vi "Bounce(LC).vi"(0 "COMPORT":refnum<visa-resource-name>="COM4", 1 "i/q_file":string, 5 "Gui(path)":path=path "C:/RageATE-Tetra/Support/TetraLabGUI", 9 "Ft directory":path=path "C:/RageATE-Tetra/Support/FieldTestApp", 11 "error in (no error)":errorcluster, 12 "Controls":T1={"ReadADC"=TRUE, "StartTest"=TRUE, "ResetRFSM"=TRUE, "FtServer"=TRUE, "CalVCO(t)"=TRUE, "Ping(t)"=TRUE, "CmdWindowHide(T)"=FALSE, "OpenNewFt(T)"=TRUE, "UseCmdFile(T)"=FALSE}, 13 "Standalone vi(t)":bool, 14 "Write i/q data file":bool) -> (2 "PingOK?(t)":bool=TRUE, 3 "P/F Bounce":bool, 6 "Data_Out":string[][](array[string])=[["Index/Ant", "Tx_Ant", "Rx_Ant", "dBFS", "MHz", "P/F_Power", "P/F_Freq"], ["1", "1", "1", "-5.663", "-6.226", "PASS", "PASS"], ["2", "2", "1", "-7.008", "-6.226", "PASS", "PASS"], ["3", "1", "2", "-6.712", "-6.226", "PASS", "PASS"], ["4", "3", "1", "-7.302", "-6.226", "PASS", "PASS"], ["5", "2", "2", "-6.729", "-6.226", "PASS", "PASS"], ["6", "4", "1", "-7.411", "-6.226", "PASS", "PASS"], ["7", "3", "2", "-6.907", "-6.226", "PASS", "PASS"], ["8", "2", "3", "-5.919", "-6.152", "PASS", "PASS"], ["9", "4", "2", "-6.829", "-6.226", "PASS", "PASS"], ["10", "3", "3", "-5.795", "-6.226", "PASS", "PASS"], ["11", "5", "2", "-7.206", "-6.226", "PASS", "PASS"], ["12", "4", "3", "-6.209", "-6.226", "PASS", "PASS"], ["13", "3", "4", "-6.316", "-6.226", "PASS", "PASS"], ["14", "5", "3", "-5.848", "-6.226", "PASS", "PASS"], ["15", "4", "4", "-6.060", "-6.226", "PASS", "PASS"], ["16", "6", "3", "-6.797", "-6.226", "PASS", "PASS"], ["17", "5", "4", "-5.983", "-6.226", "PASS", "PASS"], ["18", "7", "3", "-5.772", "-6.152", "PASS", "PASS"], ["19", "6", "4", "-5.572", "-6.226", "PASS", "PASS"], ["20", "5", "5", "-6.223", "-6.226", "PASS", "PASS"], ["21", "7", "4", "-5.813", "-6.226", "PASS", "PASS"], ["22", "6", "5", "-6.423", "-6.226", "PASS", "PASS"], ["23", "8", "4", "-5.728", "-6.226", "PASS", "PASS"], ["24", "7", "5", "-5.739", "-6.226", "PASS", "PASS"], ["25", "6", "6", "-5.901", "-6.226", "PASS", "PASS"], ["26", "8", "5", "-5.879", "-6.226", "PASS", "PASS"], ["27", "7", "6", "-5.680", "-6.226", "PASS", "PASS"], ["28", "9", "5", "-6.898", "-6.226", "PASS", "PASS"], ["29", "8", "6", "-5.680", "-6.226", "PASS", "PASS"], ["30", "10", "5", "-6.902", "-6.226", "PASS", "PASS"], ["31", "9", "6", "-6.670", "-6.226", "PASS", "PASS"], ["32", "8", "7", "-5.577", "-6.226", "PASS", "PASS"], ["33", "10", "6", "-6.776", "-6.226", "PASS", "PASS"], ["34", "9", "7", "-6.721", "-6.226", "PASS", "PASS"], ["35", "11", "6", "-7.184", "-6.226", "PASS", "PASS"], ["36", "10", "7", "-7.166", "-6.226", "PASS", "PASS"], ["37", "9", "8", "-6.669", "-6.226", "PASS", "PASS"], ["38", "11", "7", "-6.752", "-6.226", "PASS", "PASS"], ["39", "10", "8", "-6.667", "-6.226", "PASS", "PASS"], ["40", "12", "7", "-6.185", "-6.226", "PASS", "PASS"], ["41", "11", "8", "-6.673", "-6.226", "PASS", "PASS"], ["42", "12", "8", "-7.339", "-6.226", "PASS", "PASS"]], 8 "Ampl_Graph":dbl[][](graph), 10 "Freq_Graph":dbl[](graph), 15 "error out":errorcluster)   [LabVIEW 2018]
uses:
  C:/RageATE-Tetra/Support/TetraLabGUI/FieldTestClient.dll
  Support/TetraLabGUI/FieldTestClient.dll
  Tetra WAM/Tetra_Globals.vi
panel:
  in  "Tab Control":enum32{"Gui", "Tabular", "Settings"}(tab)
  out "status":string
  out "RESULT:":string
  in  "START":bool
  in  "CONT(t)":bool
  out "Elapsed Time":string caption="Elapsed Time Text"
  in  "Rev-C(T)":bool
  out "#ofBounces":i32
  out "py_comport":string=" -COM4"
  in  "ampl_lsl":dbl=-12.5 format="%#_13g"
  in  "ampl_hsl":dbl=2.5 format="%#_13g"
  out "StartTest?(P/F)":bool
  out "VcoCalibration?(T)":bool
  out "Close":bool
  out "ReadADC":bool=TRUE
  out "StartTest":bool
  out "ResetRFSM":bool
  out "FtServer":bool
  out "CalVCO(t)":bool
  out "Ping(t)":bool=TRUE
  out "CmdWindowHide(T)":bool
  out "OpenNewFt(T)":bool
  out "UseCmdFile(T)":bool
  out "hostName":string="localhost"
  out "portNum":i32=50501
  out "standard output":string="b'OK\\n\\r'\r\nDMA Length: 43008\r\nTx_1 Rx_1: {'Frequency': 'Passed', 'Power': 'Passed'}\r\nMax Value: -5.663 dBFS at -6.226 MHz\r\nTx_2 Rx_1: {'Frequency': 'Passed', 'Power': 'Passed'}\r\nMax Value: -7.008 dBFS at -6.226 MHz\r\nTx_1 Rx_2: {'Frequency': 'Passed', 'Power': 'Passed'}\r\nMax Value: -6.712 dBFS at -6.226 MHz\r\nTx_3 Rx_1: {'Frequency': 'Passed', 'Power': 'Passed'}\r\nMax Value: -7.302 dBFS at -6.226 MHz\r\nTx_2 Rx_2: {'Frequency': 'Passed', 'Power': 'Passed'}\r\nMax Value: -6.729 dBFS at -6.226 MHz\r\nTx_4 Rx_1: {'Frequency': 'Passed', 'Power': 'Passed'}\r\nMax Value: -7.411 dBFS at -6.226 MHz\r\nTx_3 Rx_2: {'Frequency': 'Passed', 'Power': 'Passed'}\r\nMax Value: -6.907 dBFS at -6.226 MHz\r\nTx_2 Rx_3: {'Frequency': 'Passed', 'Power': 'Passed'}\r\nMax Value: -5.919 dBFS at -6.152 MHz\r\nTx_4 Rx_2: {'Frequency': 'Passed', 'Power': 'Passed'}\r\nMax Value: -6.829 dBFS at -6.226 MHz\r\nTx_3 Rx_3: {'Frequency': 'Passed', 'Power': 'Passed'}\r\nMax Value: -5.795 dBFS at -6.226 MHz\r\nTx_5 Rx_2: {'Frequency': 'Passed', 'Power': 'Passed'}\r\nMax Value: -7.206 dBFS at -6.226 MHz\r\nTx_4 Rx_3: {'Frequency': 'Passed', 'Power': 'Passed'}\r\nMax Value: -6.209 dBFS at -6.226 MHz\r\nTx_3 Rx_4: {'Frequency': 'Passed', 'Power': 'Passed'}\r\nMax Value: -6.316 dBFS at -6.226 MHz\r\nTx_5 Rx_3: {'Frequency': 'Passed', 'Power': 'Passed'}\r\nMax Value: -5.848 dBFS at -6.226 MHz\r\nTx_4 Rx_4: {'Frequency': 'Passed', 'Power': 'Passed'}\r\nMax Value: -6.060 dBFS at -6.226 MHz\r\nTx_6 Rx_3: {'Frequency': 'Passed', 'Power': 'Passed'}\r\nMax Value: -6.797 dBFS at -6.226 MHz\r\nTx_5 Rx_4: {'Frequency': 'Passed', 'Power': 'Passed'}\r\nMax Value: -5.983 dBFS at -6.226 MHz\r\nTx_7 Rx_3: {'Frequency': 'Passed', 'Power': 'Passed'}\r\nMax Value: -5.772 dBFS at -6.152 MHz\r\nTx_6 Rx_4: {'Frequency': 'Passed', 'Power': 'Passed'}\r\nMax Value: -5.572 dBFS at -6.226 MHz\r\nTx_5 Rx_5: {'Frequency': 'Passed', 'Power': 'Passed'}\r\nMax Value: -6.223 dBFS at -6.226 MHz\r\nTx_7 Rx_4: {'Frequency': 'Passed', 'Power': 'Passed'}\r\nMax Value: -5.813 dBFS at -6.226 MHz\r\nTx_6 Rx_5: {'Frequency': 'Passed', 'Power': 'Passed'}\r\nMax Value: -6.423 dBFS at -6.226 MHz\r\nTx_8 Rx_4: {'Frequency': 'Passed', 'Power': 'Passed'}\r\nMax Value: -5.728 dBFS at -6.226 MHz\r\nTx_7 Rx_5: {'Frequency': 'Passed', 'Power': 'Passed'}\r\nMax Value: -5.739 dBFS at -6.226 MHz\r\nTx_6 Rx_6: {'Frequency': 'Passed', 'Power': 'Passed'}\r\nMax Value: -5.901 dBFS at -6.226 MHz\r\nTx_8 Rx_5: {'Frequency': 'Passed', 'Power': 'Passed'}\r\nMax Value: -5.879 dBFS at -6.226 MHz\r\nTx_7 Rx_6: {'Frequency': 'Passed', 'Power': 'Passed'}\r\nMax Value: -5.680 dBFS at -6.226 MHz\r\nTx_9 Rx_5: {'Frequency': 'Passed', 'Power': 'Passed'}\r\nMax Value: -6.898 dBFS at -6.226 MHz\r\nTx_8 Rx_6: {'Frequency': 'Passed', 'Power': 'Passed'}\r\nMax Value: -5.680 dBFS at -6.226 MHz\r\nTx_10 Rx_5: {'Frequency': 'Passed', 'Power': 'Passed'}\r\nMax Value: -6.902 dBFS at -6.226 MHz\r\nTx_9 Rx_6: {'Frequency': 'Passed', 'Power': 'Passed'}\r\nMax Value: -6.670 dBFS at -6.226 MHz\r\nTx_8 Rx_7: {'Frequency': 'Passed', 'Power': 'Passed'}\r\nMax Value: -5.577 dBFS at -6.226 MHz\r\nTx_10 Rx_6: {'Frequency': 'Passed', 'Power': 'Passed'}\r\nMax Value: -6.776 dBFS at -6.226 MHz\r\nTx_9 Rx_7: {'Frequency': 'Passed', 'Power': 'Passed'}\r\nMax Value: -6.721 dBFS at -6.226 MHz\r\nTx_11 Rx_6: {'Frequency': 'Passed', 'Power': 'Passed'}\r\nMax Value: -7.184 dBFS at -6.226 MHz\r\nTx_10 Rx_7: {'Frequency': 'Passed', 'Power': 'Passed'}\r\nMax Value: -7.166 dBFS at -6.226 MHz\r\nTx_9 Rx_8: {'Frequency': 'Passed', 'Power': 'Passed'}\r\nMax Value: -6.669 dBFS at -6.226 MHz\r\nTx_11 Rx_7: {'Frequency': 'Passed', 'Power': 'Passed'}\r\nMax Value: -6.752 dBFS at -6.226 MHz\r\nTx_10 Rx_8: {'Frequency': 'Passed', 'Power': 'Passed'}\r\nMax Value: -6.667 dBFS at -6.226 MHz\r\nTx_12 Rx_7: {'Frequency': 'Passed', 'Power': 'Passed'}\r\nMax Value: -6.185 dBFS at -6.226 MHz\r\nTx_11 Rx_8: {'Frequency': 'Passed', 'Power': 'Passed'}\r\nMax Value: -6.673 dBFS at -6.226 MHz\r\nTx_12 Rx_8: {'Frequency': 'Passed', 'Power': 'Passed'}\r\nMax Value: -7.339 dBFS at -6.226 MHz\r\n"
  out "standard error":string
  out "ReadADC_Command":string
  out "ref_time":dbl caption="Get Start Time (s)"
  out "AMPL(P/F)":bool
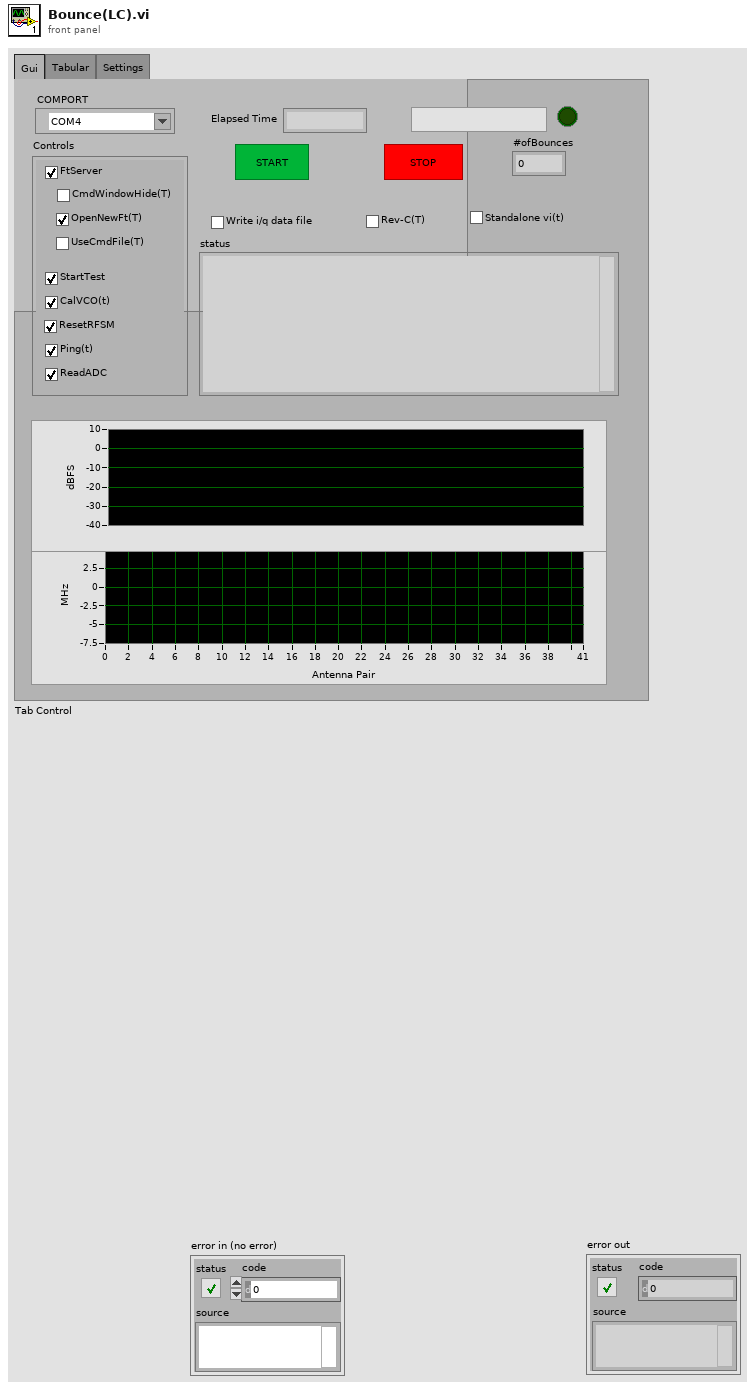
[diagram p1: front panel]
types:
  T1 = cluster{"ReadADC":bool, "StartTest":bool, "ResetRFSM":bool, "FtServer":bool, "CalVCO(t)":bool, "Ping(t)":bool, "CmdWindowHide(T)":bool, "OpenNewFt(T)":bool, "UseCmdFile(T)":bool}
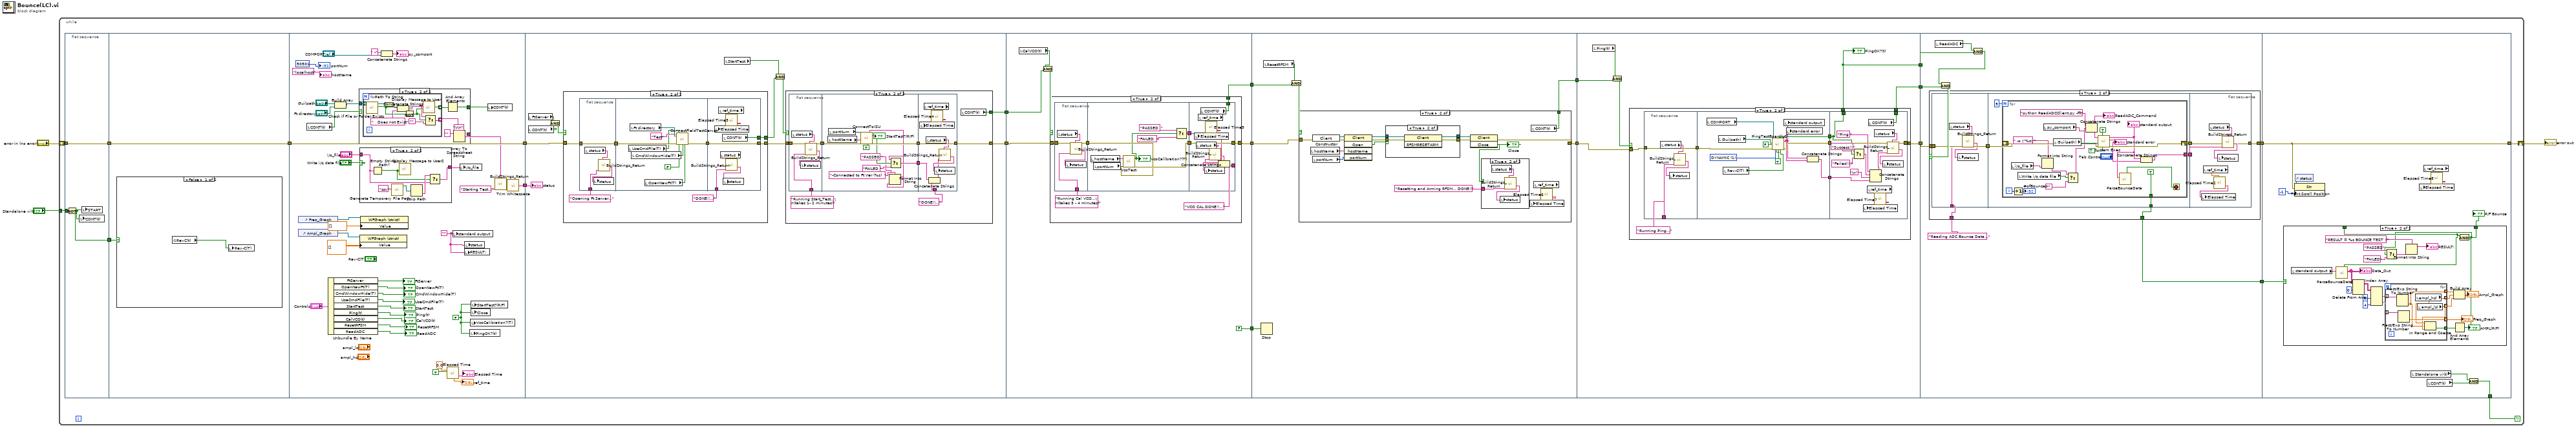
[diagram p0: block diagram]
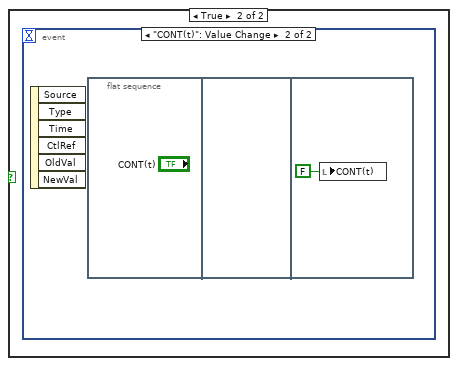
[diagram p2: hidden frame]
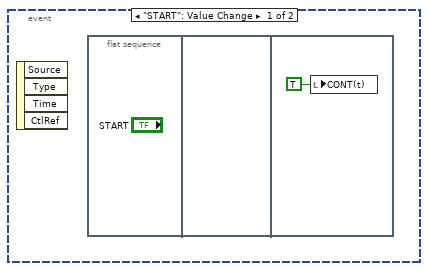
[diagram p3: hidden frame]
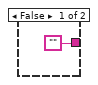
[diagram p4: hidden frame]
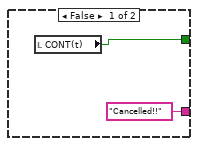
[diagram p5: hidden frame]
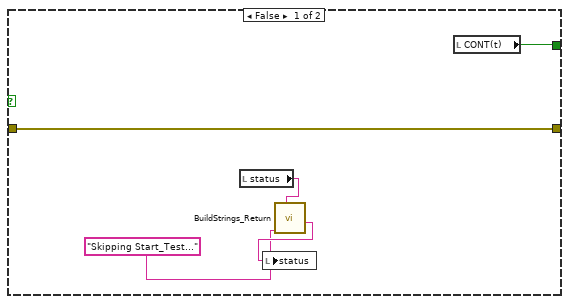
[diagram p6: hidden frame]
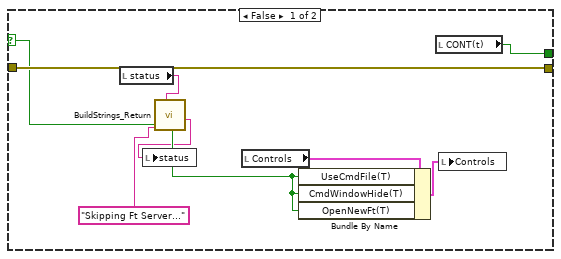
[diagram p7: hidden frame]
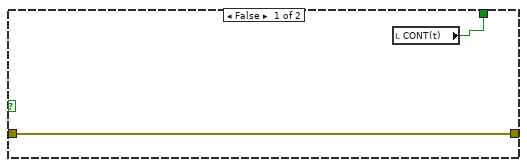
[diagram p8: hidden frame]
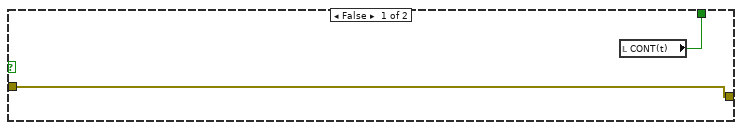
[diagram p9: hidden frame]
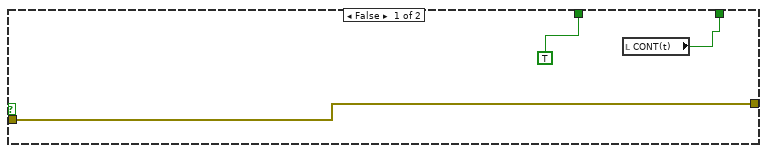
[diagram p12: hidden frame]
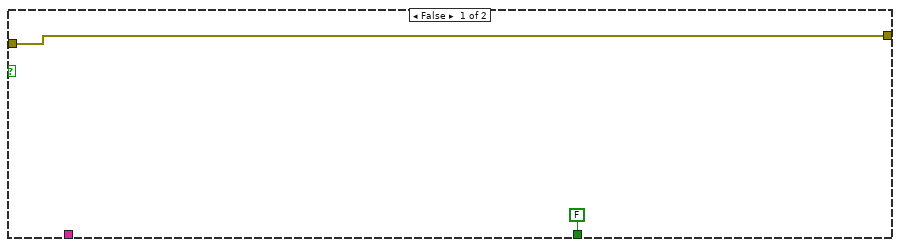
[diagram p13: hidden frame]
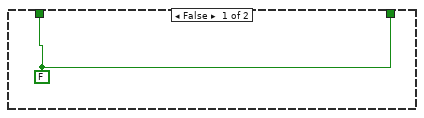
[diagram p14: hidden frame]
diagram:
  n1 = while {
    shift-right: [w14] -> w2
    shift-left: "error in (no error)" -> [w15]
    tunnel: "Standalone vi(t)" -> [w5]
    stop <- w11 continue-if-true
    n2 = flat-sequence {
      tunnel: w15 -> [w27]
      tunnel: [w27] -> w12
      tunnel: w5 -> [w25]
      tunnel: [w25] -> w4
      tunnel: [w29] -> w13
      tunnel: w12 -> [w29]
      tunnel: w4 -> [w28]
      tunnel: [w70] -> w24
      tunnel: [w61] -> w23
      tunnel: w13 -> [w70]
      tunnel: [w103] -> w22
      tunnel: w24 -> [w105]
      tunnel: w23 -> [w104]
      tunnel: [w95] -> w9
      tunnel: w22 -> [w183]
      tunnel: [w182] -> w21
      tunnel: [FALSE ("stop? (T)")] -> w10
      tunnel: w9 -> [w178]
      tunnel: [w177] -> w8
      tunnel: w21 -> [w221]
      tunnel: [w220] -> w20
      tunnel: w10 -> [w218]
      tunnel: w8 -> [w216]
      tunnel: [w215] -> w7
      tunnel: [w255] -> w18
      tunnel: w20 -> [w254]
      tunnel: [w253] -> w19
      tunnel: w7 -> [w250]
      tunnel: [w249] -> w6
      tunnel: w19 -> [w304]
      tunnel: w18 -> [w305]
      tunnel: [w306] -> w17
      tunnel: [w301] -> w16
      tunnel: w6 -> [w298]
      tunnel: [w359] -> w14
      tunnel: w17 -> [w359]
      tunnel: w16 -> [w358]
      tunnel: [w354] -> w11
      frame #0 {
        n3 = Not(x=w25) -> (.not. x?=w26:bool)
        n4 = local write "CONT(t)"(w26) -> ()
        n5 = local write "START"(w26) -> ()
      }
      frame #1 {
        n6 = case shown="False" w28 {
          frame False {
            n7 = global read "Tetra_Globals.vi" "RevC(t)"() -> (w30:bool)
            n8 = local write "Rev-C(T)"(w30) -> ()
          }
          frame True {
            n9 = event shown="[1] \"CONT(t)\": Value Change" {
              selector: _ -> [_ _]
              dyn-events: _ -> [_ _]
              timeout: _ -> [_ _]
              event "START": Value Change {
                n10 = event-data() -> ()  [unwired: 1 in, 4 out]
                n11 = flat-sequence {
                  frame #0 {
                  }
                  frame #1 {
                  }
                  frame #2 {
                    n12 = local write "CONT(t)"(TRUE ("CONT(t)")) -> ()
                  }
                }
              }
              event "CONT(t)": Value Change {
                n13 = event-data() -> ()  [unwired: 1 in, 6 out]
                n14 = flat-sequence {
                  frame #0 {
                  }
                  frame #1 {
                  }
                  frame #2 {
                    n15 = local write "CONT(t)"(FALSE ("CONT(t)")) -> ()
                  }
                }
              }
            }
          }
        }
      }
      frame #2 {
        w67 = FALSE ("StartTest?(P/F)")
        w49 = ""
        n16 = control-ref of="Ampl_Graph"() -> (w60:refnum<vi>)
        n17 = control-ref of="Freq_Graph"() -> (w59:refnum<vi>)
        n18 = local read "CONT(t)"() -> (w38:bool)
        n19 = Unbundle By Name("Controls") -> ("FtServer"=→"FtServer":bool, "OpenNewFt(T)"=→"OpenNewFt(T)":bool, "CmdWindowHide(T)"=→"CmdWindowHide(T)":bool, "UseCmdFile(T)"=→"UseCmdFile(T)":bool, "StartTest"=→"StartTest":bool, "Ping(t)"=→"Ping(t)":bool, "CalVCO(t)"=→"CalVCO(t)":bool, "ResetRFSM"=→"ResetRFSM":bool, "ReadADC"=→"ReadADC":bool)
        n20 = Build Array("Gui(path)", "Ft directory") -> (w42:path[])
        n21 = case shown="True" w38 {
          tunnel: w42 -> [_ w86]
          tunnel: [w79 w84] -> w40
          tunnel: ["Cancelled!!" ("spreadsheet string") w83] -> w39
          frame False {
            n22 = local read "CONT(t)"() -> (w79:bool)
          }
          frame True {
            n23 = for {
              tunnel: w86 -> [w94] mode=indexing
              tunnel: [w87] -> w85 mode=indexing
              tunnel: [w88] -> w82 mode=indexing
              n24 = call <vilib>:"Check if File or Folder Exists.vi"("path"=w94) -> ("file or folder exists?"=w87:bool)  [unwired: 8 in, 2 out]
              n25 = Path To String(path=w94) -> (string=w93:string)
              n26 = Concatenate Strings(w93, "   Does not Exist" ("string")) -> (w90:string)
              n27 = Not(x=w87) -> (.not. x?=w91:bool)
              n28 = call "Display Message to User"("Enable"=w91, "Message"=w90) -> ()  [unwired: 8 in, 2 out]
              n29 = Select(t=w90, s=w91, f="") -> (s? t:f=w88:string)
            }
            n30 = And Array Elements(Boolean array=w85) -> (logical AND=w84:bool)
            n31 = Array To Spreadsheet String(delimiter (Tab)="\r\n", array=w82, 3:"" ("format string")) -> (spreadsheet string=w83:string)
          }
        }
        n32 = case shown="True" "Write i/q data file" {
          tunnel: ["" w75] -> w34
          tunnel: "i/q_file" -> [_ w73]
          frame False {
          }
          frame True {
            n33 = Empty String/Path?(string/path=w73) -> (empty?=w72:bool)
            n34 = call <vilib>:"Generate Temporary File Path.vi"("Temporary File Extension (tmp)"="csv") -> ("Unique Temporary File Path"=w76:path)  [unwired: 9 in, 1 out]
            n35 = call "Display Message to User2"("Enable"=w72) -> ()  [unwired: 9 in, 2 out]
            n36 = Strip Path(path=w76) -> (name=w74:string)  [unwired: 1 out]
            n37 = Select(t=w74, s=w72, f=w73) -> (s? t:f=w75:string)
          }
        }
        n38 = property class="WFGraph (strict)"(reference=w60, "Value"=dbl[][] []) -> ()  [unwired: 1 in, 2 out]
        n39 = property class="WFGraph (strict)"(reference=w59, "Value"=dbl[] []) -> ()  [unwired: 1 in, 2 out]
        n40 = Concatenate Strings(" -" ("string"), "COMPORT") -> (→"py_comport":string)
        n41 = call "Elapsed Time"("Reset"=TRUE, "Set Start Time (s)"=0.0) -> ("Get Start Time (s)"=→"ref_time":dbl, "Elapsed Time Text"=→"Elapsed Time":string)  [unwired: 10 in, 6 out]
        n42 = local write "standard output"(w49) -> ()
        n43 = local write "i/q_file"(w34) -> ()
        n44 = local write "RESULT:"(w49) -> ()
        n45 = local write "status"(w49) -> ()
        n46 = local write "PingOK?(t)"(w67) -> ()
        n47 = local write "VcoCalibration?(T)"(w67) -> ()
        n48 = local write "StartTest?(P/F)"(w67) -> ()
        n49 = local write "Close"(w67) -> ()
        n50 = local write "CONT(t)"(w40) -> ()
        n51 = call "BuildStrings_Return.vi"("Input String"=w39, "New String"="Starting Test...") -> ("concatenated string"=w62:string)  [unwired: 7 in, 2 out]
        n52 = call <vilib>:"Trim Whitespace.vi"("string"=w62) -> ("trimmed string"=w61:string)  [unwired: 1 in]
        "hostName" <- "localhost" ("hostName")
        "portNum" <- 50501 ("portNum")
      }
      frame #3 {
        n53 = local read "FtServer"() -> (w101:bool)
        n54 = local read "CONT(t)"() -> (w99:bool)
        n55 = And(x=w101, y=w99) -> (x .and. y?=w100:bool)
        n56 = case shown="True" w100 {
          selector: w100 -> [w147 _]
          tunnel: w105 -> [w150 w157]
          tunnel: [w150 w156] -> w102
          tunnel: [w143 w151] -> w96
          frame False {
            n57 = local read "status"() -> (w146:string)
            n58 = call "BuildStrings_Return.vi"("Input String"=w146, "New String"="Skipping Ft Server...") -> ("concatenated string"=w145:string)  [unwired: 7 in, 2 out]
            n59 = local write "status"(w145) -> ()
            n60 = local read "Controls"() -> (w149:T1)
            n61 = Bundle By Name(cluster=w149, "UseCmdFile(T)"=w147, "CmdWindowHide(T)"=w147, "OpenNewFt(T)"=w147) -> (w148:T1)
            n62 = local read "CONT(t)"() -> (w143:bool)
            n63 = local write "Controls"(w148) -> ()
          }
          frame True {
            n64 = flat-sequence {
              tunnel: w157 -> [w161]
              tunnel: [w161] -> w154
              tunnel: "Opening Ft Server..." -> [w159]
              tunnel: [w168] -> w155
              tunnel: w154 -> [w169]
              tunnel: [w176] -> w156
              tunnel: w155 -> [w176]
              tunnel: "DONE!!..." -> [w174]
              tunnel: [w170] -> w151
              frame #0 {
                n65 = local read "status"() -> (w160:string)
                n66 = call "BuildStrings_Return.vi"("Input String"=w160, "New String"=w159) -> ("concatenated string"=w158:string)  [unwired: 7 in, 2 out]
                n67 = local write "status"(w158) -> ()
              }
              frame #1 {
                n68 = local read "UseCmdFile(T)"() -> (w162:bool)
                n69 = local read "Ft directory"() -> (w167:path)
                n70 = local read "CmdWindowHide(T)"() -> (w163:bool)
                n71 = local read "OpenNewFt(T)"() -> (w164:bool)
                n72 = call "ConnectFieldTestServer.vi"("FileName(.txt)"="Test", "working directory"=w167, "error in (no error)"=w169, "UseCmdFile(T)"=w162, "Skip(T)"=FALSE, "CmdWindowHide(T)"=w163, "OpenNewFt(T)"=w164) -> ("error out"=w168:errorcluster)  [unwired: 6 in, 6 out]
              }
              frame #2 {
                n73 = local read "ref_time"() -> (w171:dbl)
                n74 = local read "status"() -> (w175:string)
                n75 = local read "CONT(t)"() -> (w170:bool)
                n76 = call "Elapsed Time3"("Set Start Time (s)"=w171) -> ("Elapsed Time Text"=w172:string)  [unwired: 11 in, 7 out]
                n77 = local write "Elapsed Time"(w172) -> ()
                n78 = call "BuildStrings_Return.vi"("Input String"=w175, "New String"=w174) -> ("concatenated string"=w173:string)  [unwired: 7 in, 2 out]
                n79 = local write "status"(w173) -> ()
              }
            }
          }
        }
        n80 = local read "StartTest"() -> (w98:bool)
        n81 = And(x=w98, y=w96) -> (x .and. y?=w97:bool)
        n82 = case shown="True" w97 {
          tunnel: w102 -> [w110 w118]
          tunnel: [w110 w117] -> w103
          tunnel: [w106 w111] -> w95
          frame False {
            n83 = local read "status"() -> (w108:string)
            n84 = call "BuildStrings_Return.vi"("Input String"=w108, "New String"="Skipping Start_Test...") -> ("concatenated string"=w109:string)  [unwired: 7 in, 2 out]
            n85 = local write "status"(w109) -> ()
            n86 = local read "CONT(t)"() -> (w106:bool)
          }
          frame True {
            n87 = flat-sequence {
              tunnel: w118 -> [w122]
              tunnel: [w122] -> w116
              tunnel: "Running Start_Test...\n(takes 1- 2 minutes)" -> [w119]
              tunnel: w116 -> [w134]
              tunnel: [w133] -> w115
              tunnel: [w127] -> w112
              tunnel: [w142] -> w117
              tunnel: w115 -> [w142]
              tunnel: "DONE!!..." -> [w139]
              tunnel: w112 -> [w137]
              frame #0 {
                n88 = local read "status"() -> (w121:string)
                n89 = call "BuildStrings_Return.vi"("Input String"=w121, "New String"=w119) -> ("concatenated string"=w120:string)  [unwired: 7 in, 2 out]
                n90 = local write "status"(w120) -> ()
              }
              frame #1 {
                n91 = local read "hostName"() -> (w131:string)
                n92 = local read "portNum"() -> (w132:i32)
                n93 = call "ConnectToISU.vi"("error in (no error)"=w134, "hostName"=w131, "portNum"=w132, "RunStartTest(T)"=TRUE) -> ("StartTest?(P/F)"=w128:bool, "GetVersion"=w124:string, "error out"=w133:errorcluster)  [unwired: 11 in, 2 out]
                "StartTest?(P/F)" <- w128
                n94 = Format Into String(format string="-Connected to Ft Ver (%s)  ", initial string="PASSED ", w124) -> (resulting string=w123:string)  [unwired: 1 in, 1 out]
                n95 = Select(t=w123, s=w128, f="FAILED ") -> (s? t:f=w127:string)
              }
              frame #2 {
                n96 = local read "ref_time"() -> (w135:dbl)
                n97 = local read "status"() -> (w140:string)
                n98 = Concatenate Strings(w137, w139) -> (w138:string)
                n99 = call "Elapsed Time4"("Set Start Time (s)"=w135) -> ("Elapsed Time Text"=w136:string)  [unwired: 11 in, 7 out]
                n100 = local write "Elapsed Time"(w136) -> ()
                n101 = call "BuildStrings_Return.vi"("Input String"=w140, "New String"=w138) -> ("concatenated string"=w141:string)  [unwired: 7 in, 2 out]
                n102 = local write "status"(w141) -> ()
              }
            }
            n103 = local read "CONT(t)"() -> (w111:bool)
          }
        }
        "status" <- w104
      }
      frame #4 {
        n104 = local read "CalVCO(t)"() -> (w181:bool)
        n105 = And(x=w181, y=w178) -> (x .and. y?=w179:bool)
        n106 = case shown="True" w179 {
          tunnel: w183 -> [w185 w193]
          tunnel: [w185 w192] -> w182
          tunnel: [w184 w186] -> w177
          frame False {
            n107 = local read "CONT(t)"() -> (w184:bool)
          }
          frame True {
            n108 = flat-sequence {
              tunnel: w193 -> [w197]
              tunnel: [w197] -> w191
              tunnel: "Running Cal VCO...\n(takes 3 - 4 minutes)" -> [w194]
              tunnel: w191 -> [w202]
              tunnel: [w203] -> w190
              tunnel: [w198] -> w187
              tunnel: [w214] -> w192
              tunnel: w190 -> [w214]
              tunnel: "VCO CAL DONE!!..." -> [w211]
              tunnel: w187 -> [w209]
              tunnel: [w206] -> w186
              frame #0 {
                n109 = local read "status"() -> (w196:string)
                n110 = call "BuildStrings_Return.vi"("Input String"=w196, "New String"=w194) -> ("concatenated string"=w195:string)  [unwired: 7 in, 2 out]
                n111 = local write "status"(w195) -> ()
              }
              frame #1 {
                n112 = local read "hostName"() -> (w205:string)
                n113 = local read "portNum"() -> (w204:i32)
                n114 = call "VcoTest.vi"("error in (no error)"=w202, "hostName"=w205, "portNum"=w204) -> ("VcoCalibration?(T)"=w199:bool, "error out"=w203:errorcluster)  [unwired: 13 in, 2 out]
                "VcoCalibration?(T)" <- w199
                n115 = Select(t="PASSED  ", s=w199, f="FAILED  ") -> (s? t:f=w198:string)
              }
              frame #2 {
                n116 = local read "status"() -> (w212:string)
                n117 = local read "ref_time"() -> (w207:dbl)
                n118 = local read "CONT(t)"() -> (w206:bool)
                n119 = call "Elapsed Time5"("Set Start Time (s)"=w207) -> ("Elapsed Time Text"=w208:string)  [unwired: 11 in, 7 out]
                n120 = local write "Elapsed Time"(w208) -> ()
                n121 = Concatenate Strings(w209, w211) -> (w210:string)
                n122 = call "BuildStrings_Return.vi"("Input String"=w212, "New String"=w210) -> ("concatenated string"=w213:string)  [unwired: 7 in, 2 out]
                n123 = local write "status"(w213) -> ()
              }
            }
          }
        }
      }
      frame #5 {
        n124 = Stop(stop? (T)=w218) -> ()
        n125 = local read "ResetRFSM"() -> (w219:bool)
        n126 = And(x=w219, y=w216) -> (x .and. y?=w217:bool)
        n127 = case shown="True" w217 {
          tunnel: w221 -> [w223 w239]
          tunnel: [w223 w227] -> w220
          tunnel: [w222 w224] -> w215
          frame False {
            n128 = local read "CONT(t)"() -> (w222:bool)
          }
          frame True {
            n129 = local read "hostName"() -> (w237:string)
            n130 = constructor class="Client"(error in=w239) -> (reference out=w238:refnum<k24>, error out=w234:errorcluster)  [unwired: 2 in, 1 out]
            n131 = local read "portNum"() -> (w236:i32)
            n132 = invoke class="Client" method="Open"(reference=w238, error in=w234, "hostName"=w237, "portNum"=w236) -> (reference out=w235:refnum<k24>, error out=w233:errorcluster, "Open"=w232:bool)  [unwired: 1 in, 2 out]
            n133 = case shown="True" w232 {
              tunnel: [w244 w248] -> w230
              tunnel: w235 -> [w243 w246]
              tunnel: w233 -> [w244 w245]
              tunnel: [w243 w247] -> w231
              frame False {
              }
              frame True {
                n134 = invoke class="Client" method="RFSMRESETARM"(reference=w246, error in=w245) -> (reference out=w247:refnum<k24>, error out=w248:errorcluster)  [unwired: 1 in, 1 out]
              }
            }
            n135 = invoke class="Client" method="Close"(reference=w231, error in=w230) -> (error out=w227:errorcluster, "Close"=w228:bool)  [unwired: 1 in, 1 out]
            "Close" <- w228
            n136 = case shown="True" w228 {
              tunnel: "Resetting and Arming RFSM... DONE!!" -> [_ w240]
              frame False {
              }
              frame True {
                n137 = local read "status"() -> (w242:string)
                n138 = call "BuildStrings_Return.vi"("Input String"=w242, "New String"=w240) -> ("concatenated string"=w241:string)  [unwired: 7 in, 2 out]
                n139 = local write "status"(w241) -> ()
              }
            }
            n140 = local read "CONT(t)"() -> (w224:bool)
            n141 = local read "ref_time"() -> (w226:dbl)
            n142 = call "Elapsed Time6"("Set Start Time (s)"=w226) -> ("Elapsed Time Text"=w225:string)  [unwired: 11 in, 7 out]
            n143 = local write "Elapsed Time"(w225) -> ()
          }
        }
      }
      frame #6 {
        n144 = local read "Ping(t)"() -> (w252:bool)
        n145 = And(x=w252, y=w250) -> (x .and. y?=w251:bool)
        n146 = case shown="True" w251 {
          tunnel: [w258 w260] -> w255
          tunnel: w254 -> [w258 w267]
          tunnel: [TRUE ("OK?(t)") w262] -> w253
          tunnel: [w256 w259] -> w249
          frame False {
            n147 = local read "CONT(t)"() -> (w256:bool)
          }
          frame True {
            n148 = flat-sequence {
              tunnel: w267 -> [w271]
              tunnel: [w271] -> w265
              tunnel: "Running Ping..." -> [w268]
              tunnel: [w283] -> w266
              tunnel: w265 -> [w282]
              tunnel: [w277] -> w263
              tunnel: [w274] -> w261
              tunnel: [w297] -> w260
              tunnel: w266 -> [w297]
              tunnel: w263 -> [w294]
              tunnel: [w294] -> w262
              tunnel: w261 -> [w289]
              tunnel: [w284] -> w259
              frame #0 {
                n149 = local read "status"() -> (w269:string)
                n150 = call "BuildStrings_Return.vi"("Input String"=w269, "New String"=w268) -> ("concatenated string"=w270:string)  [unwired: 7 in, 2 out]
                n151 = local write "status"(w270) -> ()
              }
              frame #1 {
                w280 = TRUE ("ExeCommands(T)")
                w281 = 1 items=["CW", "DYNAMIC"] ("Mode Select")
                n152 = local read "COMPORT"() -> (w278:refnum<visa-resource-name>)
                n153 = local read "Gui(path)"() -> (w279:path)
                n154 = local read "Rev-C(T)"() -> (w272:bool)
                n155 = call "PingTestBoard(LC).vi"("COMPORT"=w278, "GuiDir"=w279, "GlobPaths(t)"=FALSE, "error in (no error)"=w282, "Mode Select"=w281, "Close Serial(T)"=w280, "ExeCommands(T)"=w280, "RevC(t)"=w272) -> ("standard error"=w275:string, "standard output"=w276:string, "OK?(t)"=w277:bool, "error out"=w283:errorcluster)  [unwired: 5 in, 3 out]
                n156 = local write "standard output"(w276) -> ()
                n157 = local write "standard error"(w275) -> ()
                n158 = Concatenate Strings(w276, w275) -> (w274:string)
              }
              frame #2 {
                n159 = Select(t="Success!! ", s=w294, f="Failed!! ") -> (s? t:f=w292:string)
                n160 = local read "ref_time"() -> (w285:dbl)
                n161 = local read "CONT(t)"() -> (w284:bool)
                n162 = Concatenate Strings("Ping ", w292, "\n", w289) -> (w287:string)
                n163 = local read "status"() -> (w296:string)
                n164 = call "Elapsed Time7"("Set Start Time (s)"=w285) -> ("Elapsed Time Text"=w286:string)  [unwired: 11 in, 7 out]
                n165 = local write "Elapsed Time"(w286) -> ()
                n166 = call "BuildStrings_Return.vi"("Input String"=w296, "New String"=w287) -> ("concatenated string"=w295:string)  [unwired: 7 in, 2 out]
                n167 = local write "status"(w295) -> ()
              }
            }
          }
        }
        "PingOK?(t)" <- w253
      }
      frame #7 {
        n168 = local read "ReadADC"() -> (w302:bool)
        n169 = And(x=w302, y=w304) -> (x .and. y?=w300:bool)
        n170 = And(x=w300, y=w298) -> (x .and. y?=w299:bool)
        n171 = case shown="True" w299 {
          tunnel: [w307 w312] -> w306
          tunnel: w305 -> [w307 w311]
          tunnel: "Reading ADC Bounce Data..." -> [_ w310]
          tunnel: [FALSE w309] -> w301
          frame False {
          }
          frame True {
            n172 = flat-sequence {
              tunnel: w311 -> [w319]
              tunnel: [w319] -> w315
              tunnel: w310 -> [w316]
              tunnel: w315 -> [w323]
              tunnel: [w324] -> w314
              tunnel: [w322] -> w313
              tunnel: [w321] -> w309
              tunnel: [w348] -> w312
              tunnel: w314 -> [w348]
              tunnel: w313 -> [w349]
              frame #0 {
                n173 = local read "status"() -> (w318:string)
                n174 = call "BuildStrings_Return.vi"("Input String"=w318, "New String"=w316) -> ("concatenated string"=w317:string)  [unwired: 7 in, 2 out]
                n175 = local write "status"(w317) -> ()
              }
              frame #1 {
                n176 = for {
                  N: 5 -> [_]
                  tunnel: [w343] -> w322
                  tunnel: [TRUE] -> w321
                  shift-right: [w345] -> w324
                  shift-left: w323 -> [w344]
                  i -> [w326]
                  stop <- w328 stop-if-true
                  n177 = local read "i/q_file"() -> (w331:string)
                  n178 = Increment(x=w326) -> (x+1=→"#ofBounces":i32)
                  n179 = local read "Write i/q data file"() -> (w335:bool)
                  n180 = Format Into String(format string=" -o \"%s\"", w331) -> (resulting string=w332:string)  [unwired: 2 in, 1 out]
                  n181 = local read "py_comport"() -> (w329:string)
                  n182 = local read "Gui(path)"() -> (w338:path)
                  n183 = Select(t=w332, s=w335, f="") -> (s? t:f=w330:string)
                  n184 = Concatenate Strings("python ReadADCClient.py -fft" ("command line 3"), w330, w329) -> (w337:string)
                  "ReadADC_Command" <- w337
                  n185 = call <vilib>:"System Exec.vi"("run minimized? (F)"=TRUE, "wait until completion? (T)"=TRUE, "error in (no error)"=w344, "working directory"=w338, "command line"=w337) -> ("error out"=w345:errorcluster, "standard error"=w336:string, "standard output"=w327:string)  [unwired: 3 in, 1 out]
                  "standard error" <- w336
                  "standard output" <- w327
                  n186 = call "ParseBounceData.vi"("Data_In"=w327) -> ("Passed?(T)"=w328:bool)  [unwired: 12 in, 2 out]
                  n187 = Concatenate Strings(w327, w336) -> (w343:string)
                }
              }
              frame #2 {
                n188 = local read "ref_time"() -> (w346:dbl)
                n189 = local read "status"() -> (w350:string)
                n190 = call "Elapsed Time2"("Set Start Time (s)"=w346) -> ("Elapsed Time Text"=w347:string)  [unwired: 11 in, 7 out]
                n191 = local write "Elapsed Time"(w347) -> ()
                n192 = call "BuildStrings_Return.vi"("Input String"=w350, "New String"=w349) -> ("concatenated string"=w351:string)  [unwired: 7 in, 2 out]
                n193 = local write "status"(w351) -> ()
              }
            }
          }
        }
      }
      frame #8 {
        n194 = case shown="True" w358 {
          tunnel: [w362 w364] -> _
          tunnel: [w362 w363] -> w352
          frame False {
            w362 = FALSE ("Passed?(T)")
          }
          frame True {
            n195 = local read "standard output"() -> (w384:string)
            n196 = call "ParseBounceData.vi"("Data_In"=w384) -> ("Passed?(T)"=w364:bool, "Data_Out"=w382:string[][])  [unwired: 12 in, 1 out]
            "Data_Out" <- w382
            n197 = Delete From Array(array=w382, index (row)=0) -> (array with subset deleted=w380:string[][])  [unwired: 2 in, 1 out]
            n198 = Index Array(array=w380, index (col) #1=3 ("index (col)"), index (col) #2=4 ("index (col)")) -> (element #1=w379:string[], element #2=w376:string[])  [unwired: 2 in]
            n199 = for {
              tunnel: w379 -> [w391] mode=indexing
              tunnel: [w386] -> w378 mode=indexing
              tunnel: w376 -> [w390] mode=indexing
              tunnel: [w389] -> w375 mode=indexing
              tunnel: [w388] -> w368 mode=indexing
              tunnel: [w387] -> w367 mode=indexing
              tunnel: [w385] -> w366 mode=indexing
              n200 = Fract/Exp String To Number(string=w391) -> (number=w386:dbl)  [unwired: 3 in, 1 out]
              n201 = Fract/Exp String To Number(string=w390) -> (number=w389:dbl)  [unwired: 3 in, 1 out]
              n202 = local read "ampl_hsl"() -> (w388:dbl)
              n203 = local read "ampl_lsl"() -> (w387:dbl)
              n204 = In Range and Coerce(upper limit=w388, x=w386, lower limit=w387) -> (In Range?=w385:bool)  [unwired: 1 out]
            }
            "Freq_Graph" <- w375
            n205 = Build Array(w378, w368, w367) -> (→"Ampl_Graph":dbl[][])
            n206 = And Array Elements(Boolean array=w366) -> (logical AND=w365:bool)
            "AMPL(P/F)" <- w365
            n207 = And(x=w364, y=w365) -> (x .and. y?=w363:bool)
            n208 = Select(t="PASSED", s=w363, f="FAILED") -> (s? t:f=w373:string)
            n209 = Format Into String(format string="RESULT = %s BOUNCE TEST !!", w373) -> (resulting string=→"RESULT:":string)  [unwired: 2 in, 1 out]
          }
        }
        "P/F Bounce" <- w352
        n210 = control-ref of="status"() -> (w361:refnum<vi>)
        n211 = property class="Str"(reference=w361, error in=w359, "Text.Scroll Position"=-1) -> ()  [unwired: 2 out]
        n212 = local read "Standalone vi(t)"() -> (w353:bool)
        n213 = local read "ref_time"() -> (w356:dbl)
        n214 = local read "CONT(t)"() -> (w357:bool)
        n215 = call "Elapsed Time8"("Set Start Time (s)"=w356) -> ("Elapsed Time Text"=w355:string)  [unwired: 11 in, 7 out]
        n216 = local write "Elapsed Time"(w355) -> ()
        n217 = And(x=w353, y=w357) -> (x .and. y?=w354:bool)
      }
    }
  }
  "error out" <- w2
